vi "Init KIM.vi"(8 "error in (no error)":errorcluster, 9 "Serial Number":string, 10 "reference":refnum<vi>, 11 ".NET Refnum in":refnum<k24>) -> (0 "error out":errorcluster, 1 "Position":i32, 2 "Enum":T1, 3 ".NET Refnum out":refnum<k24>)   [LabVIEW 2023]
uses:
  C:/Users/quantum/Documents/LVDAQ/UIs/TranslationStage_UI/Thorlabs.MotionControl.Controls.dll
  UIs/TranslationStage_UI/Thorlabs.MotionControl.Controls.dll
  KIM101_FSM/KIM_FSM_Control.ctl
  C:/Users/quantum/Documents/LVDAQ/UIs/TranslationStage_UI/Thorlabs.MotionControl.KCube.InertialMotorCLI.dll
  UIs/TranslationStage_UI/Thorlabs.MotionControl.KCube.InertialMotorCLI.dll
  KIM101.lvclass
  C:/Program Files/National Instruments/LabVIEW 2023/vi.lib/ActorFramework/Actor/Actor.lvclass
  C:/Users/quantum/Documents/LVDAQ/ConcreteClasses/ConcreteInstrumentClasses/KIM101/KIM101/KIM101.lvclass
  C:/Users/quantum/Documents/LVDAQ/Interfaces/InitDeinitInterface/InitDeinit/InitDeinit.lvclass
  C:/Users/quantum/Documents/LVDAQ/Interfaces/AbstractInstrumentClasses/TranslationStages_LV/TranslationStageInterface/TranslationStagesInterface.lvclass
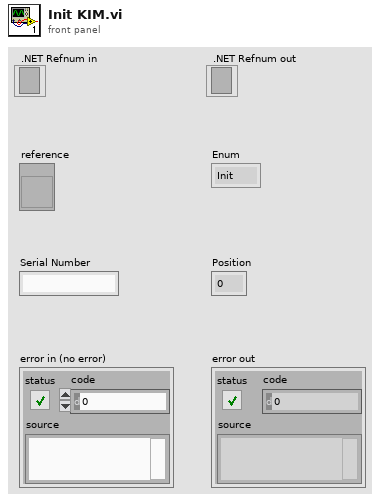
[diagram p1: front panel]
types:
  T1 = typedef "KIM_FSM_Control.ctl" = enum16{"Init", "Running", "Error", "Close"}
  T2 = cluster{"JogAcceleration":i32, "JogStepFwd":i32, "JogMode":i32, "JogRate":i32, "JogStepRev":i32}
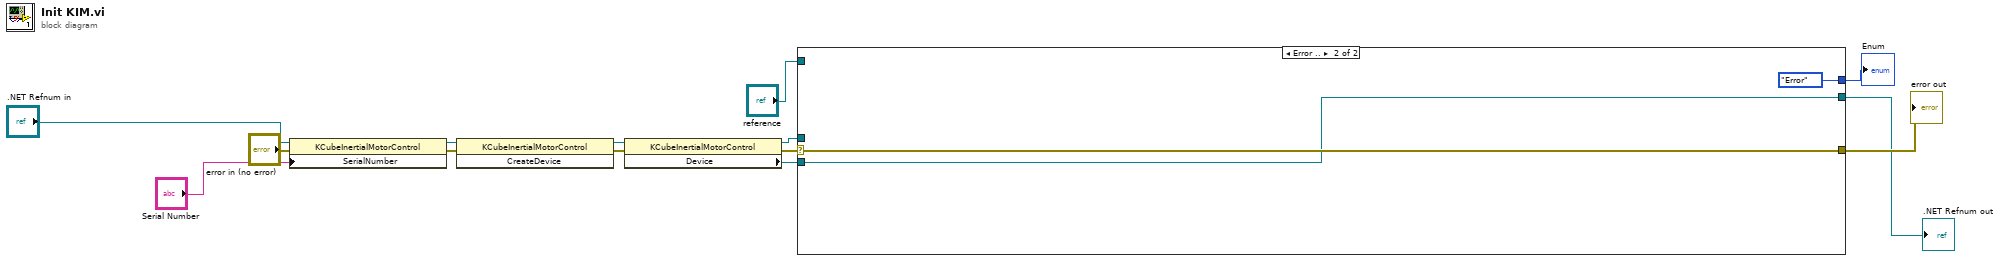
[diagram p0: block diagram]
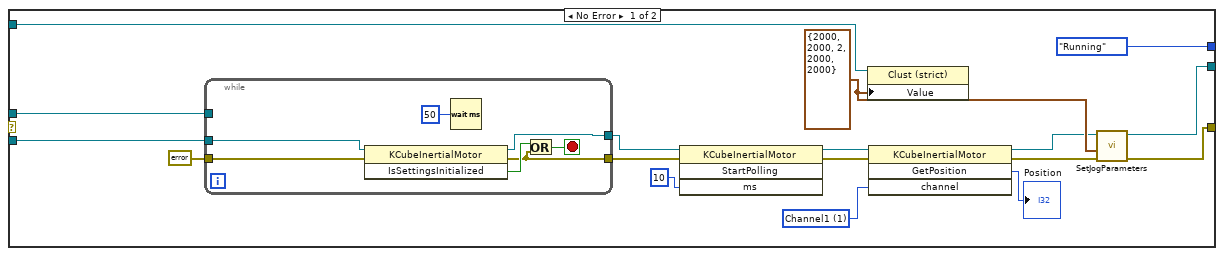
[diagram p2: hidden frame]
diagram:
  n1 = property class="KCubeInertialMotorControl"(reference=".NET Refnum in", error in="error in (no error)", "SerialNumber"="Serial Number") -> (reference out=w7:refnum<k24>, error out=w11:errorcluster)
  n2 = invoke class="KCubeInertialMotorControl" method="CreateDevice"(reference=w7, error in=w11) -> (reference out=w2:refnum<k24>, error out=w3:errorcluster)  [unwired: 1 in, 1 out]
  n3 = property class="KCubeInertialMotorControl"(reference=w2, error in=w3) -> (reference out=w13:refnum<k24>, error out=w14:errorcluster, "Device"=w12:refnum<k24>)
  n4 = case shown="Error .." w14 {
    selector: w14 -> [_ w40]
    tunnel: [KIM_FSM_Control."Running" KIM_FSM_Control."Error"] -> w4
    tunnel: [w19 w39] -> w5
    tunnel: [w20 w40] -> w6
    tunnel: w12 -> [w25 w39]
    tunnel: w13 -> [w24 _]
    tunnel: "reference" -> [w15 _]
    frame No Error {
      w18 = T2 {"JogAcceleration"=2000, "JogStepFwd"=2000, "JogMode"=2, "JogRate"=2000, "JogStepRev"=2000} ("Jog Parameters 2")
      w28 = 1 items=["Channel1"=1, "Channel2"=2, "Channel3"=3, "Channel4"=4] ("channel")
      n5 = while {
        tunnel: w25 -> [w35]
        tunnel: [w38] -> w23
        tunnel: errorcluster {"status"=FALSE, "code"=0, "source"=""} ("error in (no error)") -> [w36]
        tunnel: [w33] -> w21
        tunnel: w24 -> [_]
        stop <- w32 stop-if-true
        n6 = invoke class="KCubeInertialMotor" method="IsSettingsInitialized"(reference=w35, error in=w36) -> (reference out=w38:refnum<k24>, error out=w33:errorcluster, "IsSettingsInitialized"=w34:bool)  [unwired: 1 in]
        n7 = Wait (ms)(milliseconds to wait=u32 50) -> ()  [unwired: 1 out]
        n8 = Or(x=w34, y=w33) -> (x .or. y?=w32:bool)
      }
      n9 = invoke class="KCubeInertialMotor" method="StartPolling"(reference=w23, error in=w21, "ms"=10) -> (reference out=w30:refnum<k24>, error out=w29:errorcluster)  [unwired: 1 in, 2 out]
      n10 = property class="Clust (strict)"(reference=w15, "Value"=w18) -> ()  [unwired: 1 in, 2 out]
      n11 = invoke class="KCubeInertialMotor" method="GetPosition"(reference=w30, error in=w29, "channel"=w28) -> (reference out=w16:refnum<k24>, error out=w17:errorcluster, "GetPosition"=→"Position":i32)  [unwired: 1 in, 1 out]
      n12 = call "SetJogParameters.vi"("error in (no error)"=w17, 9:w18, "KIM101 in"=w16) -> ("error out"=w20:errorcluster, "KIM101 out"=w19:refnum<class "KIM101.lvclass">)  [unwired: 7 in]
    }
    frame Error {
    }
  }
  "error out" <- w6
  ".NET Refnum out" <- w5
  "Enum" <- w4
